vi "Write Adaptive FF settings.vi"(0 "FpgaRef5782.lvclass":refnum<class "FpgaRef5782.lvclass">, 1 "a (cavity filter)":dbl min=0.0 max=10000.0, 2 "b (cavity filter)":dbl min=0.0 max=1.0, 3 "samples to skip for inverse":i32 min=0 max=400000, 5 "Adaptive FF enabled":bool, 7 "Use inverse cavity":bool, 9 "LP filter cutoff fequency [MHz]":dbl min=0.0 max=10000.0, 11 "Adaptation factor [0-1]":dbl min=0.0 max=1.0, 12 "Samples to skip":i32 min=0 max=400000, 13 "AFF delay":i32 min=0 max=400000, 14 "PID delay":i32 min=0 max=400000) -> (4 "FpgaRef5782.lvclass":refnum<class "FpgaRef5782.lvclass">)   [LabVIEW 2018]
uses:
  FpgaRef/FpgaRef5782/FpgaRef5782.lvclass
  C:/PXIe/InProgress/source/Host/FpgaRef/FpgaRefBase/FpgaRefBase.lvclass
  FPGA/fpga_settings.ctl
  <vilib>/rvi/FXPMathLib/FxpInterpret/XNode/nifxpmath_Interpret.xnode
  FpgaRef/FpgaRefBase/FpgaRefBase.lvclass
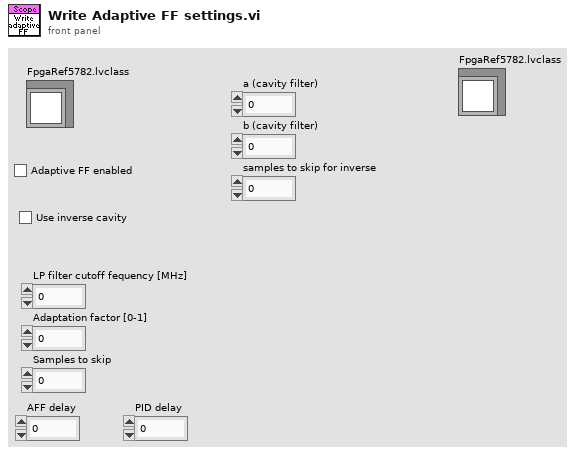
[diagram p1: front panel]
types:
  T1 = typedef "fpga_settings.ctl" = enum16{"Feedback Enable", "New FIR coeffs", "FIR shift", "Enable filter", "Set Downsample", "Downsample", "CIC Gain", "Record length", "Trigger samples", "Quiet time", "a_am", "b_am", "Use fixed delay", "fixed sin_fi", "fixed cos_fi", "Ki*Tau", "Kp", "Kd_Tau", "Fi_start", "Fi_delta", "DC_offs 0", "DC_offs 1", "DC_offs 2", "DC_offs 3", "Ki*Tau am", "Kp am", "Kd_Tau am", "Feedback AM", "Trigger delay", "Feedback delay", "Setpoint enable", "Beam enable", "Samples to acquire", "Cavity Enable", "Cavity C1", "Cavity C2", "Cavity C3", "Cavity C4", "Cavity C5", "Input delay", "Ki*Tau Q", "Kp Q", "Kd_Tau Q", "Adaptive FF enable", "Feedforward a0", "Feedforward b0", "FF src adress", "FF dest adress", "Output scale", "Input scale", "Host scale", "FF_IIR b0", "FF_IIR b1", "FF_IIR b2", "FF_IIR-a1", "FF_IIR-a2", "Enable HW trigger", "Virtual cavity", "Samples to skip", "Samples to skip 2", "Samples to skip 3", "Cavity C3_2", "Cavity C4_2", "Cavity C5_2", "Cavity C3_3", "Cavity C4_3", "Cavity C5_3", "Cavity_w0_dt", "Piezo setting", "Quench t0", "Quench tau set", "Quench enabled", "Quench reset", "PID enabled I", "PID enabled Q", "Cavity filter a", "Cavity filter b", "Disable e(n)", "FF e(n) src address", "FF first address", "FF last address", "FF PID first address", "FF PID last address"}
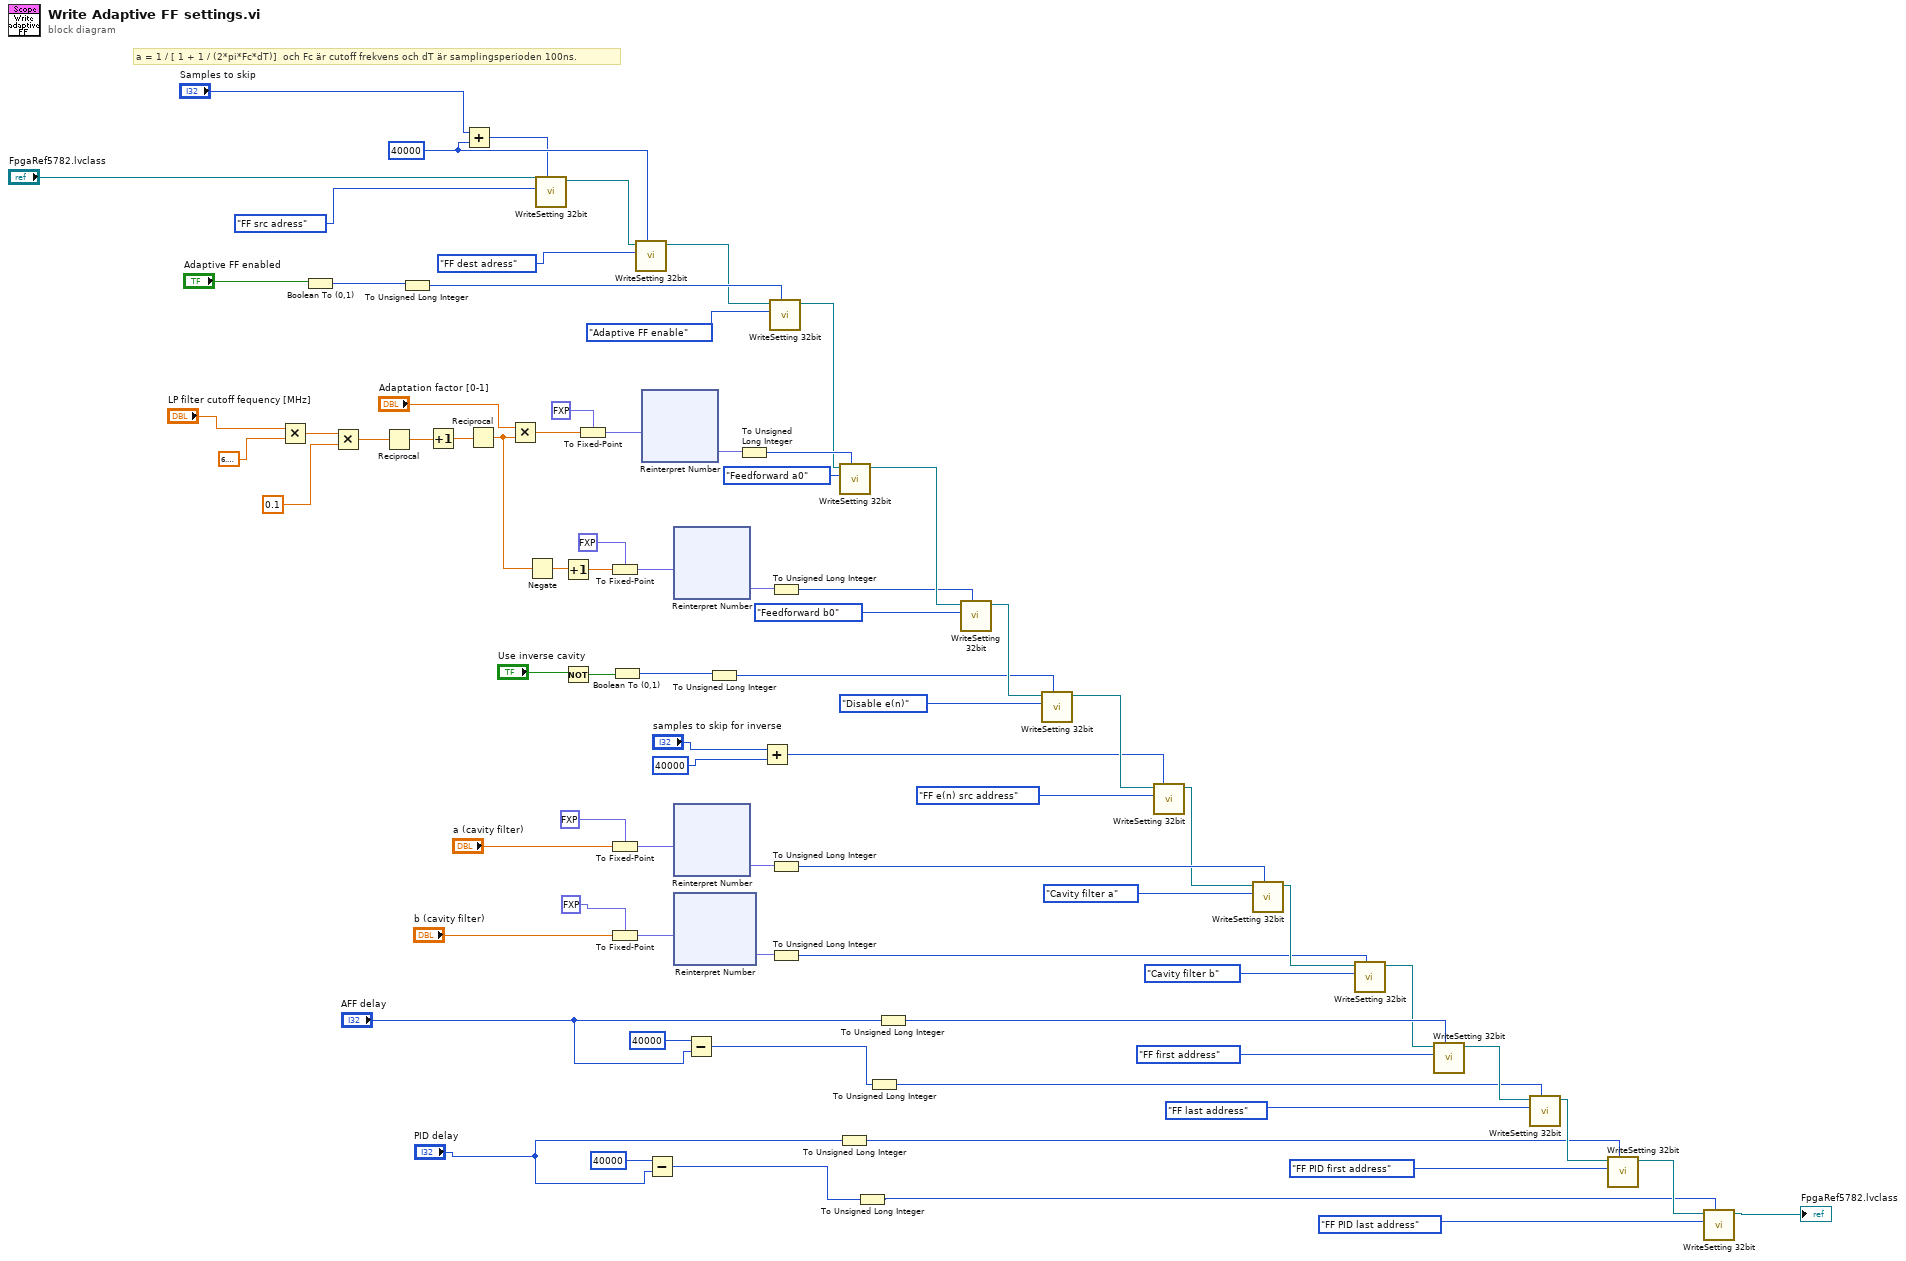
[diagram p0: block diagram]
diagram:
  w49 = u32 40000 ("value")
  # "a = 1 / [ 1 + 1 / (2*pi*Fc*dT)]  och Fc är cutoff frekvens och dT är samplingsperioden 100ns."
  n1 = Multiply(x="LP filter cutoff fequency [MHz]", y=6.283185307179586) -> (x*y=w72:dbl)
  n2 = Boolean To (0,1)(Boolean="Adaptive FF enabled") -> (0, 1=w55:i16)
  n3 = Multiply(x=w72, y=0.1) -> (x*y=w70:dbl)
  n4 = Reciprocal(x=w70) -> (1/x=w69:dbl)
  n5 = To Unsigned Long Integer(number=w55) -> (unsigned 32bit integer=w54:u32)
  n6 = Increment(x=w69) -> (x+1=w68:dbl)
  n7 = Add(x="Samples to skip", y=w49) -> (x+y=w47:u32)
  n8 = Reciprocal(x=w68) -> (1/x=w66:dbl)
  n9 = Multiply(x="Adaptation factor [0-1]", y=w66) -> (x*y=w60:dbl)
  n10 = Negate(x=w66) -> (-x=w65:dbl)
  n11 = call "WriteSetting 32bit.vi"("value"=w47, "FPGA Setting"=fpga_settings."FF src adress", "FpgaRefBase in"="FpgaRef5782.lvclass") -> ("FpgaRefBase out"=w51:refnum<class "FpgaRef5782.lvclass">)  [unwired: 7 in, 1 out]
  n12 = Increment(x=w65) -> (x+1=w59:dbl)
  n13 = Not(x="Use inverse cavity") -> (.not. x?=w40:bool)
  n14 = To Fixed-Point(fixed-point type=fxp<+/-,32,2> 0.0 ("x"), number=w60) -> (fixed-point=w78:fxp<+/-,32,2>)
  n15 = To Fixed-Point(fixed-point type=fxp<+/-,32,2> 0.0 ("x"), number=w59) -> (fixed-point=w62:fxp<+/-,32,2>)
  n16 = To Fixed-Point(fixed-point type=fxp<+/-,32,4> 0.0 ("x"), number="a (cavity filter)") -> (fixed-point=w33:fxp<+/-,32,4>)
  n17 = To Fixed-Point(fixed-point type=fxp<+/-,32,17> 0.0 ("x"), number="b (cavity filter)") -> (fixed-point=w32:fxp<+/-,32,17>)
  n18 = Boolean To (0,1)(Boolean=w40) -> (0, 1=w44:i16)
  n19 = call "WriteSetting 32bit.vi"("value"=w49, "FPGA Setting"=fpga_settings."FF dest adress", "FpgaRefBase in"=w51) -> ("FpgaRefBase out"=w53:refnum<class "FpgaRef5782.lvclass">)  [unwired: 7 in, 1 out]
  n20 = xnode "Reinterpret Number"("x"=w78) -> ("y"=w79:fxp<+,32,32>)
  n21 = Subtract(x=40000 ("value"), y="PID delay") -> (x-y=w10:i32)
  n22 = xnode "Reinterpret Number"("x"=w62) -> ("y"=w61:fxp<+,32,32>)
  n23 = xnode "Reinterpret Number"("x"=w33) -> ("y"=w34:fxp<+,32,32>)
  n24 = xnode "Reinterpret Number"("x"=w32) -> ("y"=w31:fxp<+,32,32>)
  n25 = Subtract(x=40000 ("value"), y="AFF delay") -> (x-y=w15:i32)
  n26 = To Unsigned Long Integer(number=w44) -> (unsigned 32bit integer=w43:u32)
  n27 = To Unsigned Long Integer(number=w79) -> (unsigned 32bit integer=w76:u32)
  n28 = Add(x="samples to skip for inverse", y=u32 40000 ("value")) -> (x+y=w35:u32)
  n29 = call "WriteSetting 32bit.vi"("value"=w54, "FPGA Setting"=fpga_settings."Adaptive FF enable", "FpgaRefBase in"=w53) -> ("FpgaRefBase out"=w57:refnum<class "FpgaRef5782.lvclass">)  [unwired: 7 in, 1 out]
  n30 = To Unsigned Long Integer(number=w61) -> (unsigned 32bit integer=w46:u32)
  n31 = To Unsigned Long Integer(number=w34) -> (unsigned 32bit integer=w28:u32)
  n32 = To Unsigned Long Integer(number=w31) -> (unsigned 32bit integer=w24:u32)
  n33 = To Unsigned Long Integer(number="PID delay") -> (unsigned 32bit integer=w2:u32)
  n34 = call "WriteSetting 32bit.vi"("value"=w76, "FPGA Setting"=fpga_settings."Feedforward a0", "FpgaRefBase in"=w57) -> ("FpgaRefBase out"=w58:refnum<class "FpgaRef5782.lvclass">)  [unwired: 7 in, 1 out]
  n35 = To Unsigned Long Integer(number=w10) -> (unsigned 32bit integer=w1:u32)
  n36 = To Unsigned Long Integer(number=w15) -> (unsigned 32bit integer=w12:u32)
  n37 = To Unsigned Long Integer(number="AFF delay") -> (unsigned 32bit integer=w16:u32)
  n38 = call "WriteSetting 32bit.vi"("value"=w46, "FPGA Setting"=fpga_settings."Feedforward b0", "FpgaRefBase in"=w58) -> ("FpgaRefBase out"=w45:refnum<class "FpgaRef5782.lvclass">)  [unwired: 7 in, 1 out]
  n39 = call "WriteSetting 32bit.vi"("value"=w43, "FPGA Setting"=fpga_settings."Disable e(n)", "FpgaRefBase in"=w45) -> ("FpgaRefBase out"=w38:refnum<class "FpgaRef5782.lvclass">)  [unwired: 7 in, 1 out]
  n40 = call "WriteSetting 32bit.vi"("value"=w35, "FPGA Setting"=fpga_settings."FF e(n) src address", "FpgaRefBase in"=w38) -> ("FpgaRefBase out"=w27:refnum<class "FpgaRef5782.lvclass">)  [unwired: 7 in, 1 out]
  n41 = call "WriteSetting 32bit.vi"("value"=w28, "FPGA Setting"=fpga_settings."Cavity filter a", "FpgaRefBase in"=w27) -> ("FpgaRefBase out"=w25:refnum<class "FpgaRef5782.lvclass">)  [unwired: 7 in, 1 out]
  n42 = call "WriteSetting 32bit.vi"("value"=w24, "FPGA Setting"=fpga_settings."Cavity filter b", "FpgaRefBase in"=w25) -> ("FpgaRefBase out"=w14:refnum<class "FpgaRef5782.lvclass">)  [unwired: 7 in, 1 out]
  n43 = call "WriteSetting 32bit.vi"("value"=w16, "FPGA Setting"=fpga_settings."FF first address", "FpgaRefBase in"=w14) -> ("FpgaRefBase out"=w13:refnum<class "FpgaRef5782.lvclass">)  [unwired: 7 in, 1 out]
  n44 = call "WriteSetting 32bit.vi"("value"=w12, "FPGA Setting"=fpga_settings."FF last address", "FpgaRefBase in"=w13) -> ("FpgaRefBase out"=w4:refnum<class "FpgaRef5782.lvclass">)  [unwired: 7 in, 1 out]
  n45 = call "WriteSetting 32bit.vi"("value"=w2, "FPGA Setting"=fpga_settings."FF PID first address", "FpgaRefBase in"=w4) -> ("FpgaRefBase out"=w6:refnum<class "FpgaRef5782.lvclass">)  [unwired: 7 in, 1 out]
  n46 = call "WriteSetting 32bit.vi"("value"=w1, "FPGA Setting"=fpga_settings."FF PID last address", "FpgaRefBase in"=w6) -> ("FpgaRefBase out"=→"FpgaRef5782.lvclass":refnum<class "FpgaRef5782.lvclass">)  [unwired: 7 in, 1 out]
